vi "hadamard基矢.vi"() -> ()   [LabVIEW 2016]
uses:
  <vilib>/Analysis/7linalg.llb/Create Special Real Matrix.vi
  <vilib>/Analysis/Matrix/Numeric/Conversions/Matrix To Array - RM.vi
  <vilib>/Analysis/Matrix/Numeric/Conversions/Array To Matrix - RA2.vi
  <vilib>/Analysis/Matrix/Numeric/Multiply/Multiply - RM,RM.vi
  <vilib>/Analysis/NI_AALPro.lvlib
  <vilib>/Analysis/Matrix/NI_Matrix.lvlib
panel:
  out "Numeric 2":i32
  out "show":dbl[][](graph)
  out "Numeric":i32
  out "Array":dbl[][](array[numeric])
  out "read":u32[][](graph)
  in  "path to JPEG file":path
  out "Real 2D Array":dbl[][](array[numeric])
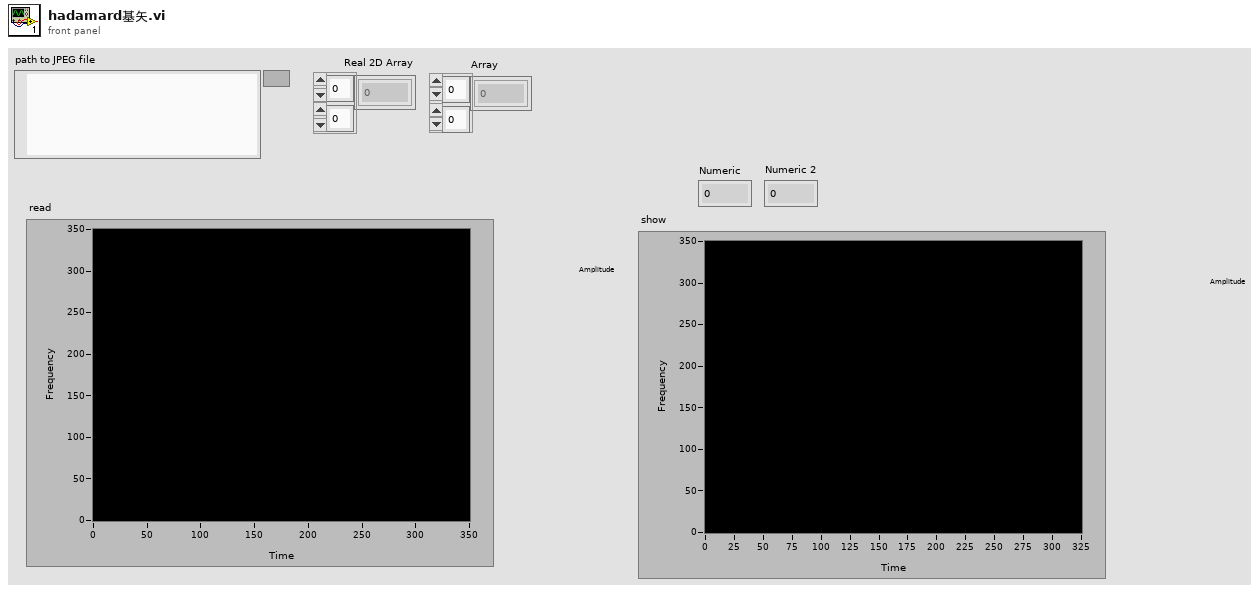
[diagram p1: front panel]
types:
  T1 = typedef "imagedata.ctl" = cluster{"image type":i32, "image depth":i32, "image":u8[], "mask":u8[], "colors":u32[], "Rectangle":cluster{"left":i16, "top":i16, "right":i16, "bottom":i16}}
  T2 = typedef "NI_Matrix.lvlib/RealMatrix.ctl" = dbl[][]
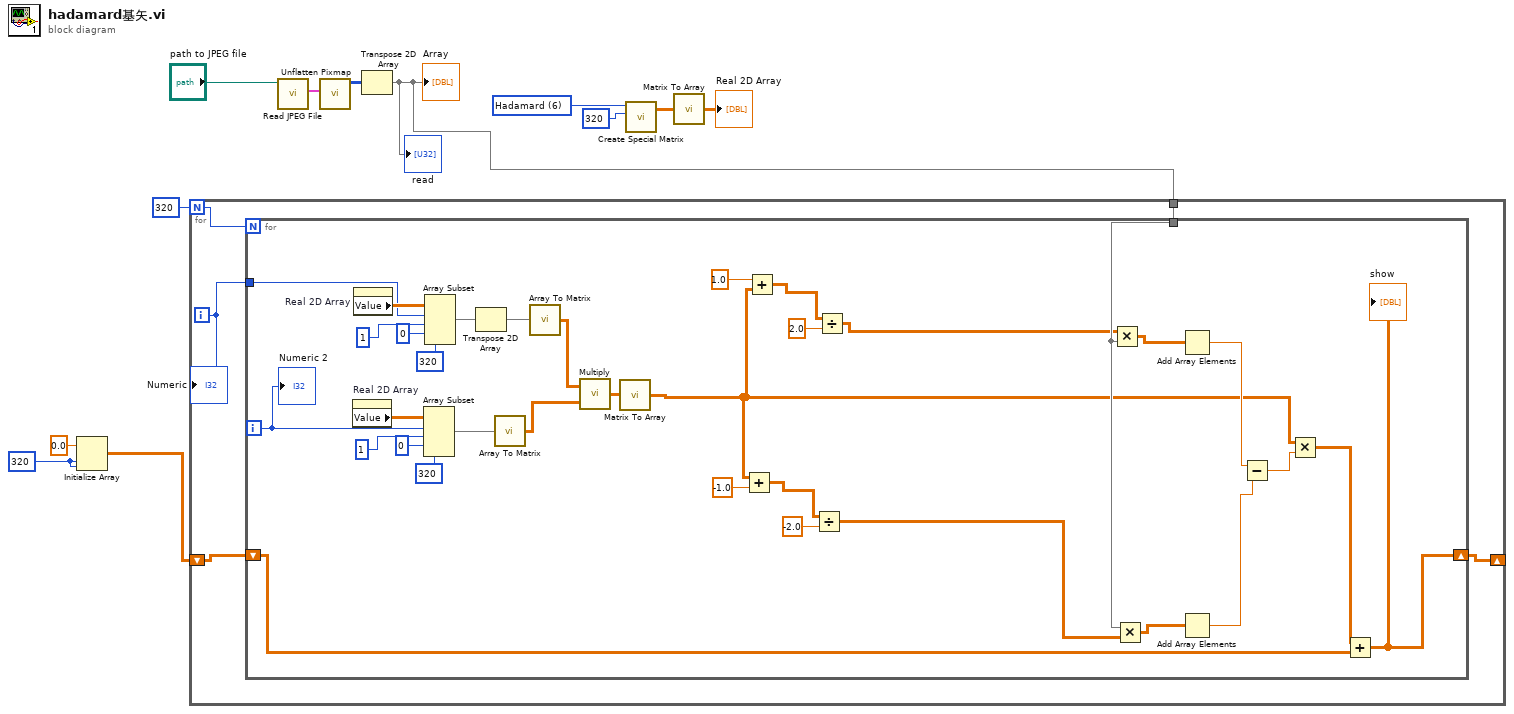
[diagram p0: block diagram]
diagram:
  w3 = 320 ("dimension size")
  w12 = 6 items=["Identity", "Diagonal", "Toeplitz", "Vandermonde", "Companion", "Hankel", "Hadamard", "Wilkinson", "Hilbert", "Inverse Hilbert", "Rosser", "Pascal"] ("matrix type")
  n1 = Initialize Array(0.0 ("element"), w3, w3) -> (w2:dbl[][])
  n2 = call <vilib>:"Read JPEG File.vi"("path to JPEG file"="path to JPEG file") -> ("image data"=w8:T1)  [unwired: 8 in, 2 out]
  n3 = call <vilib>:"Unflatten Pixmap.vi"("image data"=w8) -> ("24-bit pixmap"=w6:u32[][])  [unwired: 4 in, 6 out]
  n4 = Transpose 2D Array(2D array=w6) -> (transposed array=w1:u32[][])
  "read" <- w1
  "Array" <- w1
  n5 = for {
    N: 320 -> [w17]
    shift-right: [w15] -> _
    shift-left: w2 -> [w14]
    tunnel: w1 -> [w13]
    i -> [w16]
    n6 = for {
      N: w17 -> [_]
      tunnel: w16 -> [w43]
      shift-right: [w33] -> w15
      shift-left: w14 -> [w34]
      tunnel: w13 -> [w31]
      i -> [w32]
      n7 = property on="Real 2D Array" class="Arr (strict)"() -> ("Value"=w46:dbl[][])  [unwired: 2 in, 2 out]
      n8 = property on="Real 2D Array" class="Arr (strict)"() -> ("Value"=w49:dbl[][])  [unwired: 2 in, 2 out]
      n9 = Array Subset(array=w46, index (row)=w32, length (row)=1 ("index"), index (col)=0 ("index"), length (col)=320 ("length")) -> (w40:dbl[][])
      n10 = Array Subset(array=w49, index (row)=w43, length (row)=1 ("index"), index (col)=0 ("index"), length (col)=320 ("length")) -> (w42:dbl[][])
      n11 = Transpose 2D Array(2D array=w42) -> (transposed array=w41:dbl[][])
      n12 = call-poly <vilib>:"Array To Matrix.vi"("Real 2D Array"=w40) -> ("Real Matrix"=w38:T2)
      n13 = call-poly <vilib>:"Array To Matrix.vi"("Real 2D Array"=w41) -> ("Real Matrix"=w39:T2)
      n14 = call-poly <vilib>:"Multiply.vi"("Real Matrix B"=w38, "Real Matrix A"=w39) -> ("A * B"=w37:T2)
      n15 = call-poly <vilib>:"Matrix To Array.vi"("Real Matrix"=w37) -> ("Real 2D Array"=w18:dbl[][])
      n16 = Add(x=w18, y=-1.0) -> (x+y=w26:dbl[][])
      n17 = Add(x=1.0 ("y"), y=w18) -> (x+y=w30:dbl[][])
      n18 = Divide(x=w26, y=-2.0) -> (x/y=w23:dbl[][])
      n19 = Divide(x=w30, y=2.0) -> (x/y=w24:dbl[][])
      n20 = Multiply(x=w24, y=w31) -> (x*y=w35:dbl[][])
      n21 = Multiply(x=w31, y=w23) -> (x*y=w36:dbl[][])
      n22 = Add Array Elements(numeric array=w35) -> (sum=w22:dbl)
      n23 = Add Array Elements(numeric array=w36) -> (sum=w21:dbl)
      n24 = Subtract(x=w22, y=w21) -> (x-y=w20:dbl)
      n25 = Multiply(x=w18, y=w20) -> (x*y=w19:dbl[][])
      n26 = Add(x=w19, y=w34) -> (x+y=w33:dbl[][])
      "show" <- w33
      "Numeric 2" <- w32
    }
    "Numeric" <- w16
  }
  n27 = call-poly <vilib>:"Create Special Matrix.vi"("matrix type"=w12, "matrix size"=320) -> ("Special Matrix"=w10:T2)  [unwired: 3 in, 1 out]
  n28 = call-poly <vilib>:"Matrix To Array.vi"("Real Matrix"=w10) -> ("Real 2D Array"=→"Real 2D Array":dbl[][])
